vi "GetFont.vi"(7 "Scale":sgl=1.0, 8 "error in (no error)":errorcluster, 11 "Font(Arial,14pts,Regular)":T1={"FontName"="Arial", "Size(Pts)"=14.0, "Style"=enum."Regular"}) -> (0 "error out":errorcluster, 3 "Font":refnum<k24>)   [LabVIEW 2020, in "LcPictureBox.lvclass"]
uses:
  LcPictureBox.lvclass
  System.Drawing
  Font.ctl
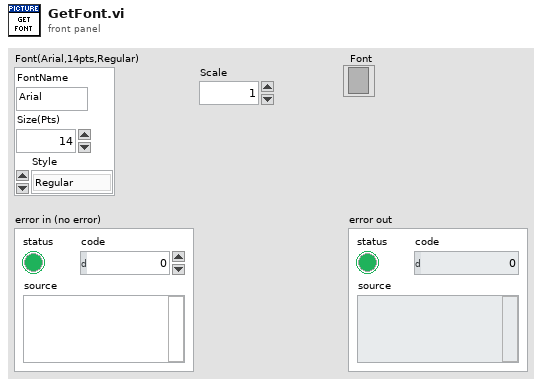
[diagram p1: front panel]
types:
  T1 = typedef "LcPictureBox.lvclass/Font.ctl" = cluster{"FontName":string, "Size(Pts)":dbl, "Style":enum16{"Regular", "Bold", "Italic", "Underline", "Strikeout"}}
  T2 = enum16{"Regular", "Bold", "Italic", "Underline", "Strikeout"}
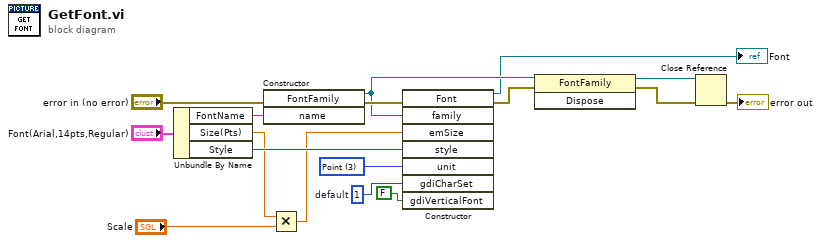
[diagram p0: block diagram]
diagram:
  w10 = 3 items=["World", "Display", "Pixel", "Point", "Inch", "Document", "Millimeter"] ("unit")
  w9 = u8 1  # default
  n1 = Unbundle By Name("Font(Arial,14pts,Regular)") -> ("FontName"=w15:string, "Size(Pts)"=w2:dbl, "Style"=w16:T2)
  n2 = constructor class="FontFamily"(error in="error in (no error)", "name"=w15) -> (reference out=w8:refnum<k24>, error out=w12:errorcluster)  [unwired: 2 in, 2 out]
  n3 = Multiply(x=w2, y="Scale") -> (x*y=w1:dbl)
  n4 = constructor class="Font"(error in=w12, "family"=w8, "emSize"=w1, "style"=w16, "unit"=w10, "gdiCharSet"=w9, "gdiVerticalFont"=FALSE) -> (reference out=→"Font":refnum<k24>, error out=w6:errorcluster)  [unwired: 2 in, 7 out]
  n5 = invoke class="FontFamily" method="Dispose"(reference=w8, error in=w6) -> (reference out=w7:refnum<k24>, error out=w5:errorcluster)  [unwired: 1 in, 1 out]
  n6 = Close Reference(reference=w7, error in (no error)=w5) -> (error out=→"error out":errorcluster)
